vi "myRIO_BRig_Host_parse_dataTrial__trim_minTrial.vi"(8 "input_minTrial":i32, 10 "input_idx":i32, 11 "input_array":i32[][](array[numeric])) -> (3 "output_cluster":cluster{i32[], i32[]})   [LabVIEW 2014]
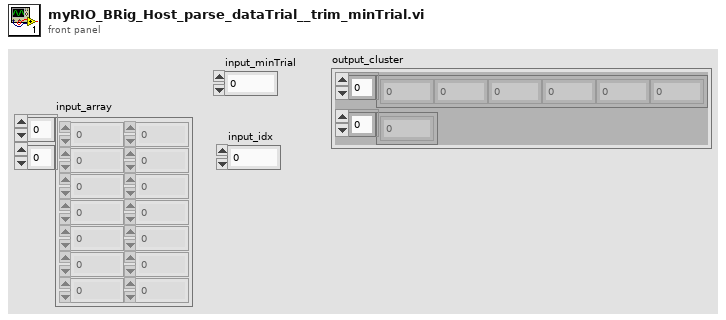
[diagram p1: front panel]
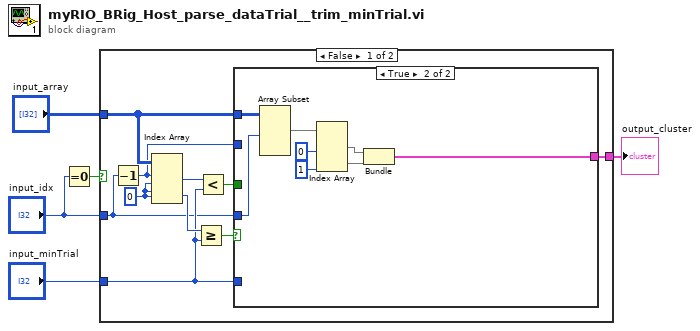
[diagram p0: block diagram]
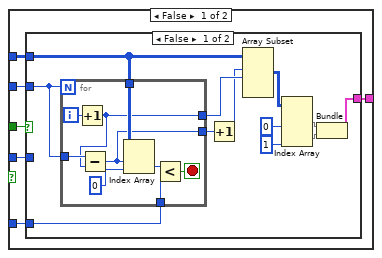
[diagram p2: hidden frame]
diagram:
  n1 = Equal To 0?(x="input_idx") -> (x = 0?=w5:bool)
  n2 = case shown="False" w5 {
    tunnel: "input_idx" -> [w7 _]
    tunnel: "input_array" -> [w11 _]
    tunnel: "input_minTrial" -> [w10 _]
    tunnel: [w9 _] -> w1
    frame False {
      w14 = 0 ("disabled index (col)")
      n3 = Decrement(x=w7) -> (x-1=w6:i32)
      n4 = Index Array(array=w11, index (row) #1=w6, index (col) #1=w14, index (row) #2=w14, index (col) #2=w14) -> (element #1=w15:i32, element #2=w13:i32)
      n5 = Greater Or Equal?(x=w13, y=w10) -> (x >= y?=w12:bool)
      n6 = Less?(x=w15, y=w10) -> (x < y?=w8:bool)
      n7 = case shown="True" w12 {
        tunnel: w11 -> [w20 w45]
        tunnel: w10 -> [w19 _]
        tunnel: [w16 w44] -> w9
        tunnel: w8 -> [w21 _]
        tunnel: w7 -> [w18 w43]
        tunnel: w6 -> [w17 _]
        frame False {
          n8 = case shown="False" w21 {
            tunnel: w20 -> [w31 _]
            tunnel: w19 -> [w33 _]
            tunnel: w18 -> [_ _]
            tunnel: w17 -> [w32 _]
            tunnel: [w22 _] -> w16
            frame False {
              n9 = for {
                N: w32 -> [_]
                tunnel: w31 -> [w41]
                tunnel: w33 -> [w39]
                tunnel: w32 -> [w37]
                tunnel: [w35] -> w30
                tunnel: [w34] -> w29
                i -> [w36]
                stop <- w38 stop-if-true
                n10 = Increment(x=w36) -> (x+1=w35:i32)
                n11 = Subtract(x=w37, y=w35) -> (x-y=w34:i32)
                n12 = Index Array(array=w41, index (row)=w34, index (col)=0) -> (element=w40:i32)
                n13 = Less?(x=w40, y=w39) -> (x < y?=w38:bool)
              }
              n14 = Increment(x=w29) -> (x+1=w28:i32)
              n15 = Array Subset(array=w31, index (row)=w28, length (row)=w30) -> (w25:i32[][])  [unwired: 2 in]
              n16 = Index Array(array=w25, index (col) #1=0 ("disabled index (col)"), index (col) #2=1 ("index (col)")) -> (element #1=w24:i32[], element #2=w23:i32[])  [unwired: 2 in]
              n17 = Bundle(w24, w23) -> (w22:cluster{i32[], i32[]})  [unwired: 1 in]
            }
            frame True {
            }
          }
        }
        frame True {
          n18 = Array Subset(array=w45, length (row)=w43) -> (w50:i32[][])  [unwired: 3 in]
          n19 = Index Array(array=w50, index (col) #1=0 ("disabled index (col)"), index (col) #2=1 ("index (col)")) -> (element #1=w47:i32[], element #2=w46:i32[])  [unwired: 2 in]
          n20 = Bundle(w47, w46) -> (w44:cluster{i32[], i32[]})  [unwired: 1 in]
        }
      }
    }
    frame True {
    }
  }
  "output_cluster" <- w1
